vi "Auto Trader_Automated.vi"() -> ()   [LabVIEW 2018]
panel:
  in  "Radius":string
  in  "Post Code":string
  out "Full Lobby":string[][](array[string])
  in  "Pages to Pull":i32
  in  "Number Of Pulls":i32
  out "Max Price Limit":i32
  out "Min Price Limit":i32
  out "All Cheapest Vehicle":string[][](array[string])
  out "Cheapest Vehicle":string[][](array[string])
  out "Iteration":i32
  out "Min Ranking":dbl
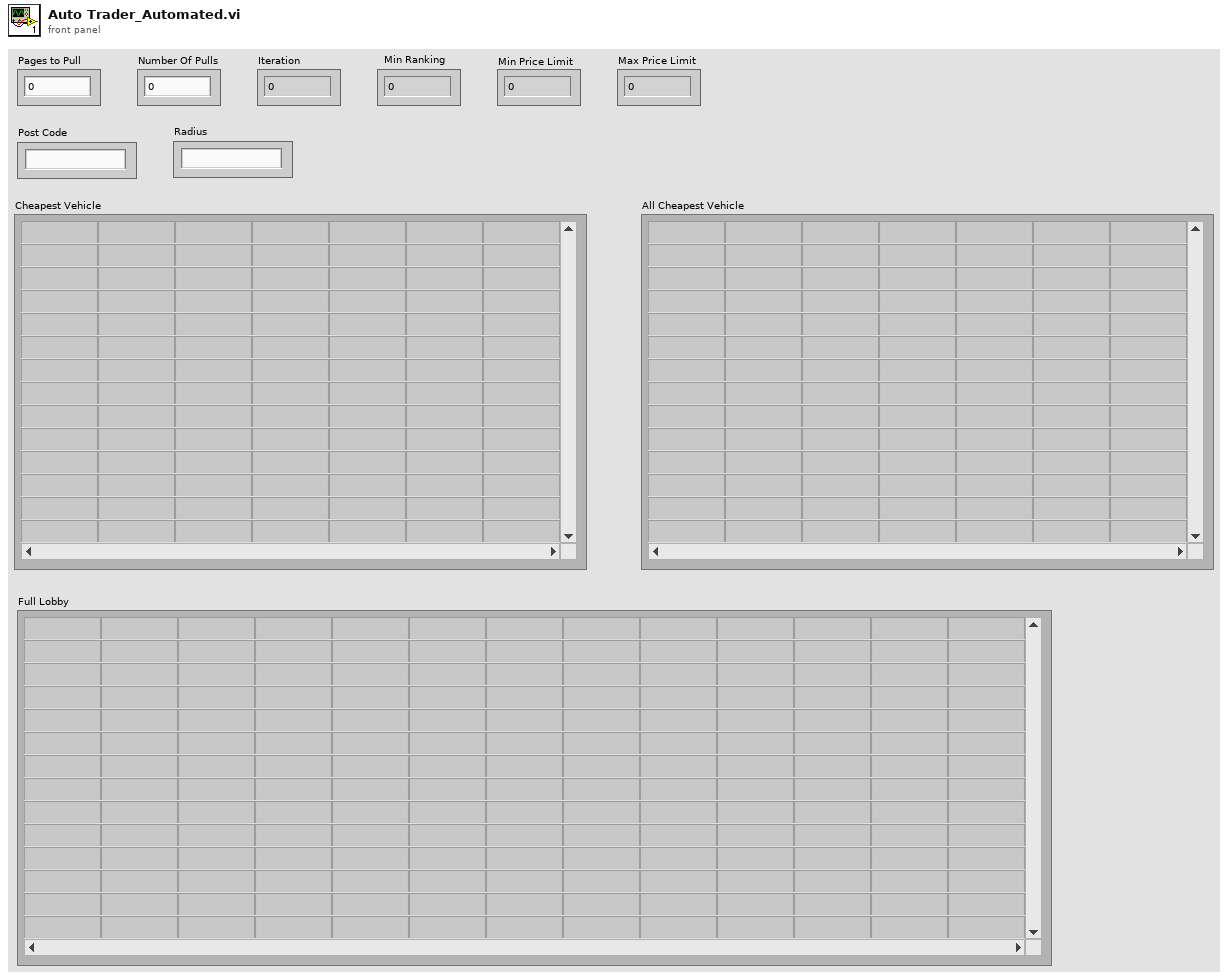
[diagram p1: front panel]
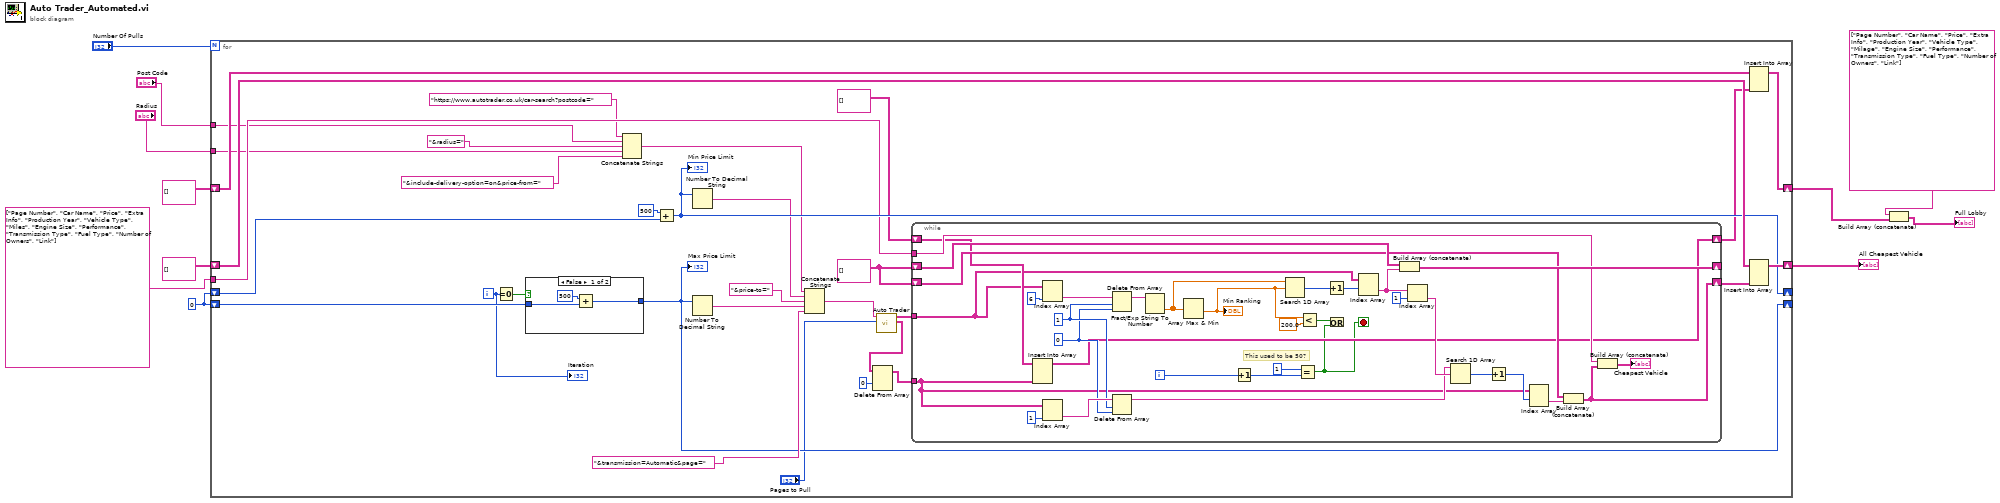
[diagram p0: block diagram]
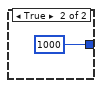
[diagram p2: hidden frame]
diagram:
  w6 = 0
  n1 = for {
    N: "Number Of Pulls" -> [_]
    shift-right: [w41] -> w9
    shift-left: string[][] [] -> [w40]
    shift-right: [w37] -> _
    shift-left: w6 -> [w38]
    shift-right: [w26] -> _
    shift-left: w6 -> [w25]
    tunnel: string[] ["Page Number", "Car Name", "Price", "Extra Info", "Production Year", "Vehicle Type", "Miles", "Engine Size", "Performance", "Transmission Type", "Fuel Type", "Number of Owners", "Link"] -> [w32]
    shift-right: [w29] -> w2
    shift-left: string[][] [] -> [w28]
    tunnel: "Post Code" -> [w20]
    tunnel: "Radius" -> [w18]
    i -> [w15]
    w43 = string[][] []
    n2 = Equal To 0?(x=w15) -> (x = 0?=w27:bool)
    n3 = case shown="False" w27 {
      tunnel: w25 -> [w46 _]
      tunnel: [w44 1000] -> w26
      frame False {
        n4 = Add(x=500, y=w46) -> (x+y=w44:i32)
      }
      frame True {
      }
    }
    "Max Price Limit" <- w26
    n5 = Concatenate Strings("https://www.autotrader.co.uk/car-search?postcode=", w20, "&radius=", w18, "&include-delivery-option=on&price-from=") -> (w16:string)
    n6 = Add(x=500, y=w38) -> (x+y=w37:i32)
    "Min Price Limit" <- w37
    n7 = Number To Decimal String(number=w37) -> (decimal integer string=w36:string)  [unwired: 1 in]
    n8 = Number To Decimal String(number=w26) -> (decimal integer string=w34:string)  [unwired: 1 in]
    n9 = Concatenate Strings(w16, w36, "&price-to=", w34, "&transmission=Automatic&page=") -> (w23:string)
    n10 = call "Auto Trader.vi"("Pages to Pull"="Pages to Pull", "Link"=w23) -> ("Pulled Cars"=w14:string[][], "Car Information"=w22:string[][])  [unwired: 7 in]
    n11 = Delete From Array(array=w14, index (row)=0) -> (array with subset deleted=w12:string[][])  [unwired: 2 in, 1 out]
    n12 = while {
      shift-right: [w78] -> _
      shift-left: w43 -> [w77]
      shift-right: [w56] -> w42
      shift-left: w43 -> [w71]
      tunnel: w32 -> [w55]
      shift-right: [w53] -> w30
      shift-left: string[][] [] -> [w52]
      tunnel: w12 -> [w51]
      tunnel: w22 -> [w50]
      i -> [w58]
      stop <- w48 stop-if-true
      w67 = 0 ("index")
      w68 = 1 ("length")
      # "This used to be 50?"
      n13 = Insert Into Array(array=w52, new element=w51) -> (w53:string[][])  [unwired: 2 in]
      n14 = Index Array(array=w50, index (col)=6 ("disabled index (col)")) -> (element=w75:string[])  [unwired: 1 in]
      n15 = Index Array(array=w51, index (col)=1 ("disabled index (col)")) -> (element=w69:string[])  [unwired: 1 in]
      n16 = Delete From Array(array=w75, length=w68, index=w67) -> (array with subset deleted=w74:string[])  [unwired: 1 out]
      n17 = Delete From Array(array=w69, length=w68, index=w67) -> (array with subset deleted=w63:string[])  [unwired: 1 out]
      n18 = Fract/Exp String To Number(string=w74) -> (number=w79:dbl[])  [unwired: 3 in, 1 out]
      n19 = Array Max & Min(array=w79) -> (min value=w76:dbl)  [unwired: 3 out]
      "Min Ranking" <- w76
      n20 = Increment(x=w58) -> (x+1=w59:i32)
      n21 = Search 1D Array(1D array=w79, element=w76) -> (index of element=w73:i32)  [unwired: 1 in]
      n22 = Equal?(x=1, y=w59) -> (x = y?=w48:bool)
      n23 = Less?(x=w76, y=200.0) -> (x < y?=w49:bool)
      n24 = Increment(x=w73) -> (x+1=w72:i32)
      n25 = Or(x=w49, y=w48) -> ()  [unwired: 1 out]
      n26 = Index Array(array=w50, index (row)=w72) -> (element=w62:string[])  [unwired: 1 in]
      n27 = Build Array (concatenate)(w77, w62) -> (w78:string[][])
      n28 = Index Array(array=w62, index=1) -> (element=w64:string)
      n29 = Search 1D Array(1D array=w63, element=w64) -> (index of element=w61:i32)  [unwired: 1 in]
      n30 = Increment(x=w61) -> (x+1=w60:i32)
      n31 = Index Array(array=w51, index (row)=w60) -> (element=w66:string[])  [unwired: 1 in]
      n32 = Build Array (concatenate)(w71, w66) -> (w56:string[][])
      n33 = Build Array (concatenate)(w55, w56) -> (→"Cheapest Vehicle":string[][])
    }
    n34 = Insert Into Array(array=w28, new element=w30) -> (w29:string[][])  [unwired: 2 in]
    n35 = Insert Into Array(array=w40, new element=w42) -> (w41:string[][])  [unwired: 2 in]
    "Iteration" <- w15
  }
  "All Cheapest Vehicle" <- w9
  n36 = Build Array (concatenate)(string[] ["Page Number", "Car Name", "Price", "Extra Info", "Production Year", "Vehicle Type", "Milage", "Engine Size", "Performance", "Transmission Type", "Fuel Type", "Number of Owners", "Link"], w2) -> (→"Full Lobby":string[][])
